vi "Distance from Home.vi"(8 "error in (no error)":errorcluster, 11 "Motors with Encoders in":refnum<class "Motors with Encoders.lvclass">) -> (0 "error out":errorcluster, 3 "Motors with Encoders out":refnum<class "Motors with Encoders.lvclass">)   [LabVIEW 2014, in "Motors with Encoders.lvlib" / "Motors with Encoders.lvclass"]
uses:
  Motors with Encoders.lvclass
  Motors with Encoders.lvclass/Motors with Encoders.ctl
panel:
  out "Distance From Home":dbl
  out "Revolutions From Home":dbl
  out "Counts from Home - After De-Quad":dbl
  out "Counts From Home Before De-Quad":u32
  out "Distance Per Rev":dbl
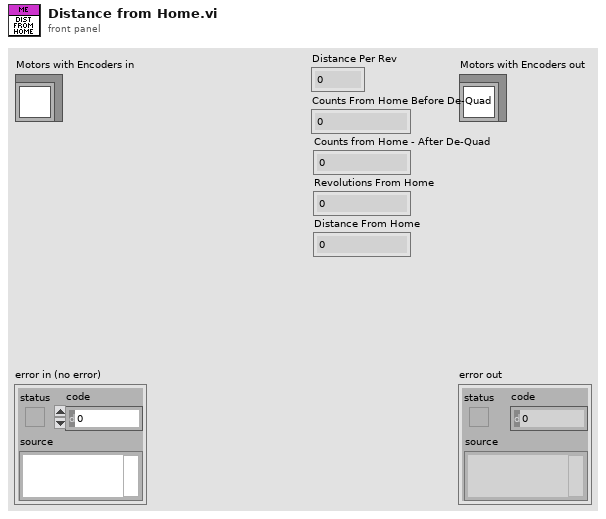
[diagram p1: front panel]
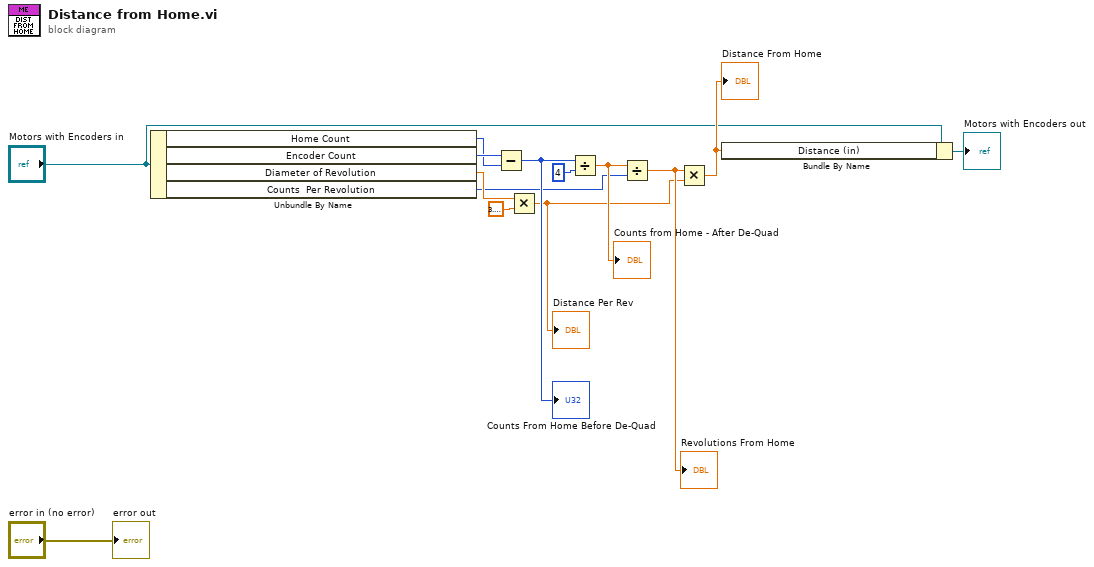
[diagram p0: block diagram]
diagram:
  n1 = Unbundle By Name("Motors with Encoders in") -> ("Home Count"=w10:i64, "Encoder Count"=w11:i64, "Diameter of Revolution"=w13:dbl, "Counts  Per Revolution"=w6:u32)
  n2 = Subtract(x=w11, y=w10) -> (x-y=w9:i64)
  "Counts From Home Before De-Quad" <- w9
  n3 = Multiply(x=w13, y=3.141592653589793) -> (x*y=w4:dbl)
  "Distance Per Rev" <- w4
  n4 = Divide(x=w9, y=u32 4) -> (x/y=w7:dbl)
  "Counts from Home - After De-Quad" <- w7
  n5 = Divide(x=w7, y=w6) -> (x/y=w5:dbl)
  "Revolutions From Home" <- w5
  n6 = Multiply(x=w5, y=w4) -> (x*y=w3:dbl)
  "Distance From Home" <- w3
  n7 = Bundle By Name(cluster="Motors with Encoders in", "Distance (in)"=w3) -> (→"Motors with Encoders out":refnum<class "Motors with Encoders.lvclass">)
  "error out" <- "error in (no error)"
